vi "HatchHook.vi"(8 "error in":errorcluster, 11 "ClusterIN":T1={"Drive Forward Input "=0.0, "Drive Twist Input"=0.0, "Drive Output"=0.0, "Drivetwist Output"=0.0, "Left Joystick Buttons"=[FALSE, FALSE, FALSE, FALSE, FALSE, FALSE, FALSE, FALSE, FALSE, FALSE, FALSE, FALSE], "Left Joystick Axis"=[-0.047244094488188976, 0.007874015748031496, -0.0, 0.12598425196850394], "Right Joystick Axis"=[0.0, -0.007874015748031496, 0.0, -1.0], "Right Joystick Button"=[FALSE, FALSE, FALSE, FALSE, FALSE, FALSE, FALSE, FALSE, FALSE, FALSE, FALSE, FALSE], "Arm Encoder"=-2.0, "Left Drive Encoder"=0.0, "Right Drive Encoder"=-1054.0, "Gyro Angle "=66.181640625, "Arm Joystick Output  "=-0.003937007874015748, "Line Follower L, C, R "=[TRUE, TRUE, TRUE], "Line follow?"=FALSE, " Climb Solenoid"=FALSE, "Wrist Encoder Count"=0.0, "Wrist Joystick Output"=0.0, "Ball Encoder Count"=0.0, "Ball Output"=0.0, "Climb Encoder"=0.0, "Climb Motor Output"=0.0, " Hatch Solenoid"=FALSE, "Arm Setpoint "=6.0, "Wrist Setpoint "=0.0, "Arm Joystick Enabled?"=FALSE, "Wrist Joystick Enabled"=FALSE, "Vision String"="0, 0, 0, 0, 0, 0", "Left Joystick POVs"=[-1]}) -> (0 "error out":errorcluster, 3 "ClusterOUT":T1={"Drive Forward Input "=0.0, "Drive Twist Input"=0.0, "Drive Output"=0.0, "Drivetwist Output"=0.0, "Left Joystick Buttons"=[FALSE, FALSE, FALSE, FALSE, FALSE, FALSE, FALSE, FALSE, FALSE, FALSE, FALSE, FALSE], "Left Joystick Axis"=[-0.047244094488188976, 0.007874015748031496, -0.0, 0.12598425196850394], "Right Joystick Axis"=[0.0, -0.007874015748031496, 0.0, -1.0], "Right Joystick Button"=[FALSE, FALSE, FALSE, FALSE, FALSE, FALSE, FALSE, FALSE, FALSE, FALSE, FALSE, FALSE], "Arm Encoder"=-2.0, "Left Drive Encoder"=0.0, "Right Drive Encoder"=-1054.0, "Gyro Angle "=66.181640625, "Arm Joystick Output  "=-0.003937007874015748, "Line Follower L, C, R "=[TRUE, TRUE, TRUE], "Line follow?"=FALSE, " Climb Solenoid"=FALSE, "Wrist Encoder Count"=0.0, "Wrist Joystick Output"=0.0, "Ball Encoder Count"=0.0, "Ball Output"=0.0, "Climb Encoder"=0.0, "Climb Motor Output"=0.0, " Hatch Solenoid"=FALSE, "Arm Setpoint "=6.0, "Wrist Setpoint "=0.0, "Arm Joystick Enabled?"=FALSE, "Wrist Joystick Enabled"=FALSE, "Vision String"="0, 0, 0, 0, 0, 0", "Left Joystick POVs"=[-1]})   [LabVIEW 2018]
uses:
  TypeDefs/Teleop Data Cluster.ctl
  TypeDefs/Joystick Buttons.ctl
  <vilib>/ptbypt/NI_PtbyPt.lvlib
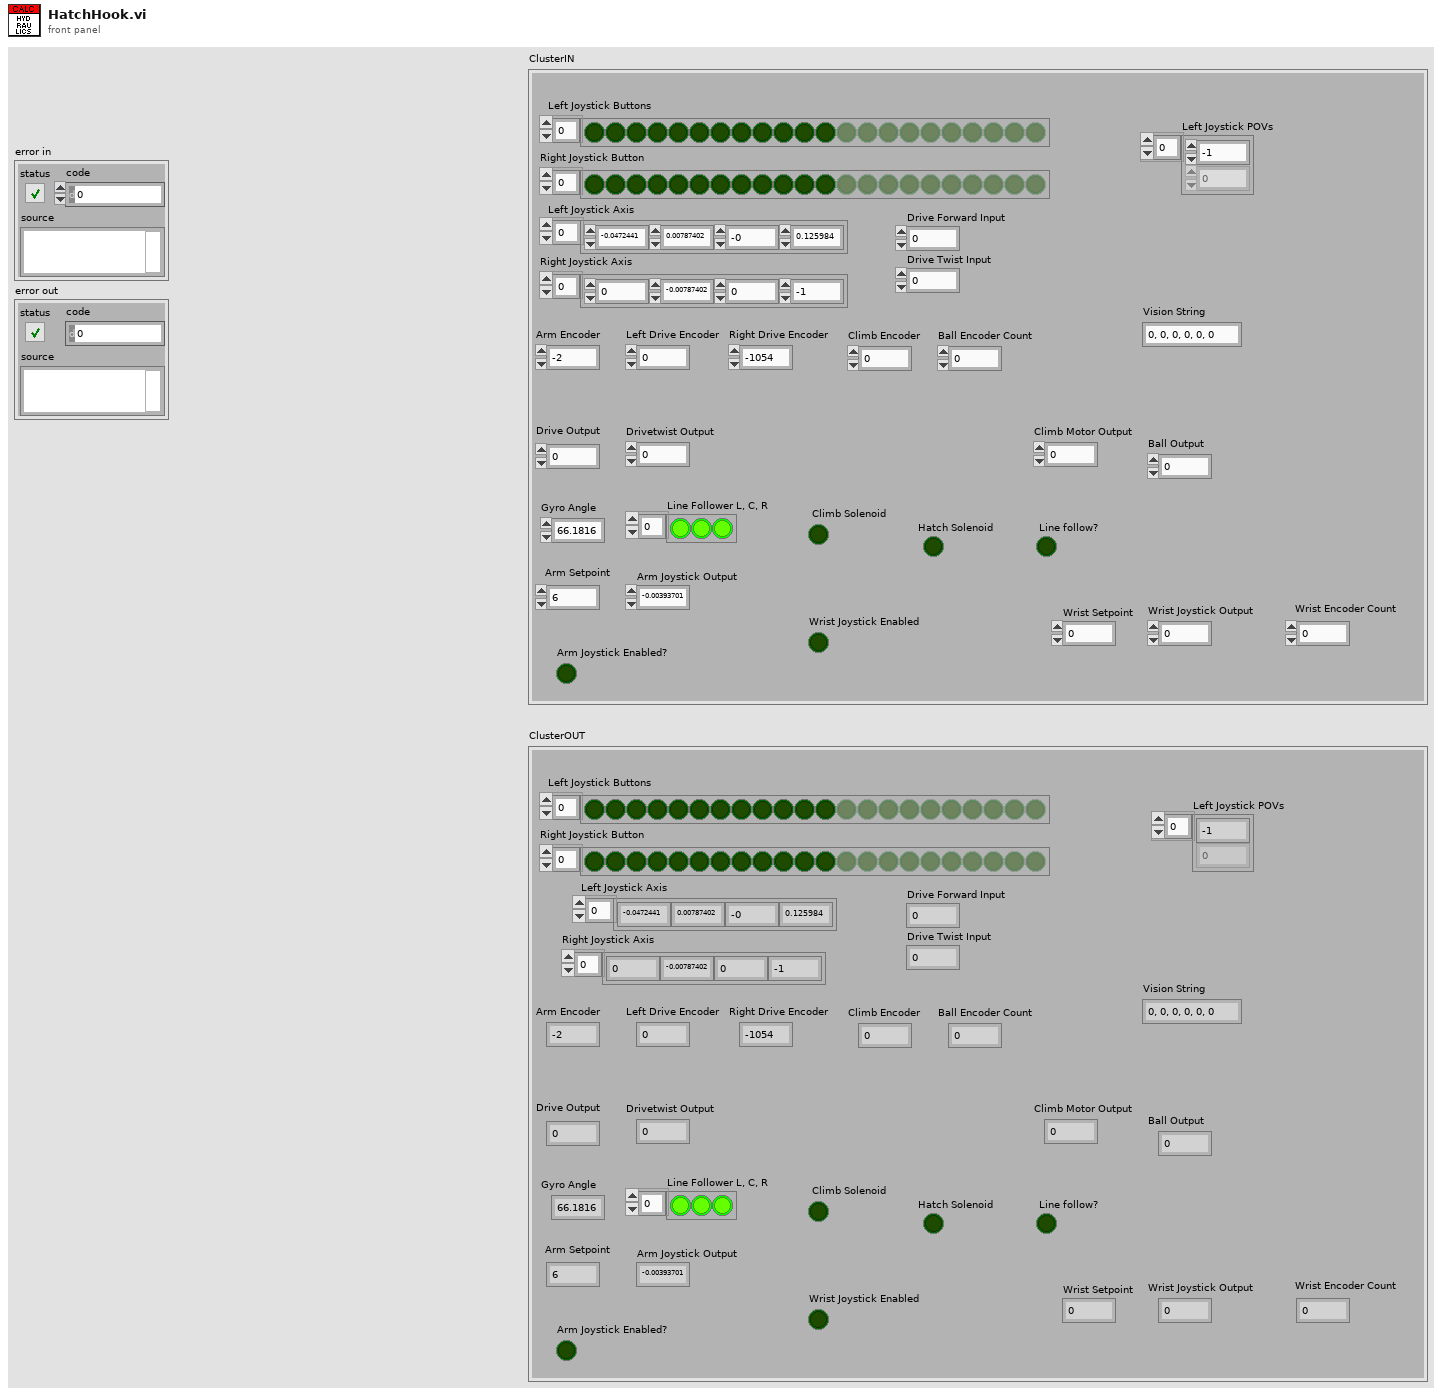
[diagram p1: front panel]
types:
  T1 = typedef "Teleop Data Cluster.ctl" = cluster{"Drive Forward Input ":dbl, "Drive Twist Input":dbl, "Drive Output":dbl, "Drivetwist Output":dbl, "Left Joystick Buttons":bool[], "Left Joystick Axis":dbl[], "Right Joystick Axis":dbl[], "Right Joystick Button":bool[], "Arm Encoder":dbl, "Left Drive Encoder":dbl, "Right Drive Encoder":dbl, "Gyro Angle ":dbl, "Arm Joystick Output  ":dbl, "Line Follower L, C, R ":bool[], "Line follow?":bool, " Climb Solenoid":bool, "Wrist Encoder Count":dbl, "Wrist Joystick Output":dbl, "Ball Encoder Count":dbl, "Ball Output":dbl, "Climb Encoder":dbl, "Climb Motor Output":dbl, " Hatch Solenoid":bool, "Arm Setpoint ":dbl, "Wrist Setpoint ":dbl, "Arm Joystick Enabled?":bool, "Wrist Joystick Enabled":bool, "Vision String":string, "Left Joystick POVs":i16[]}
  T2 = typedef "Joystick Buttons.ctl" = enum16{"Trigger", "Thumb", "Top 3", "Top 4", "Top 5", "Top 6", "Bottom 7", "Bottom 8", "Bottom 9", "Bottom 10", "Bottom 11", "Bottom 12"}
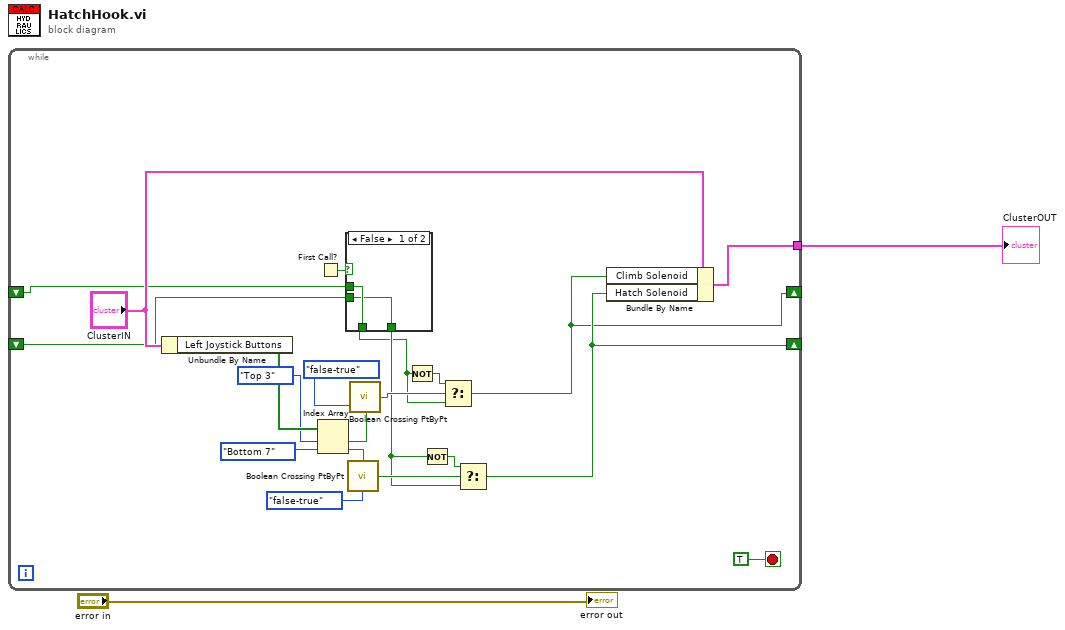
[diagram p0: block diagram]
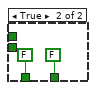
[diagram p2: hidden frame]
diagram:
  n1 = while {
    tunnel: [w20] -> w2
    shift-right: [w6] -> _
    shift-left: _ -> [w3]
    shift-right: [w5] -> _
    shift-left: _ -> [w4]
    stop <- TRUE stop-if-true
    n2 = Unbundle By Name("ClusterIN") -> ("Left Joystick Buttons"=w23:bool[])
    n3 = First Call?() -> (First Call?: T/F=w7:bool)
    n4 = Index Array(array=w23, index #1=Joystick_Buttons."Top 3" ("Enum"), index #2=Joystick_Buttons."Bottom 7" ("Enum")) -> (element #1=w18:bool, element #2=w15:bool)
    n5 = case shown="False" w7 {
      tunnel: [w24 FALSE] -> w9
      tunnel: [w25 FALSE] -> w8
      tunnel: w4 -> [w25 _]
      tunnel: w3 -> [w24 _]
      frame False {
      }
      frame True {
      }
    }
    n6 = call <vilib>:"Boolean Crossing PtByPt.vi"("direction"=enum16{"either", "false-true", "true-false"}."false-true", "input"=w15) -> ("crossing"=w10:bool)  [unwired: 1 in]
    n7 = call <vilib>:"Boolean Crossing PtByPt.vi"("direction"=enum16{"either", "false-true", "true-false"}."false-true", "input"=w18) -> ("crossing"=w13:bool)  [unwired: 1 in]
    n8 = Not(x=w8) -> (.not. x?=w12:bool)
    n9 = Not(x=w9) -> (.not. x?=w11:bool)
    n10 = Select(t=w12, s=w13, f=w8) -> (s? t:f=w5:bool)
    n11 = Select(t=w11, s=w10, f=w9) -> (s? t:f=w6:bool)
    n12 = Bundle By Name(cluster="ClusterIN", "Climb Solenoid"=w5, "Hatch Solenoid"=w6) -> (w20:T1)
  }
  "ClusterOUT" <- w2
  "error out" <- "error in"
